vi "newTestStandStringVariable.vi"(0 "Engine Reference":refnum<k7>, 5 "Sequence File Ref":refnum<k7>, 7 "Variable Name":string="Locals.temp", 9 "Variable Value":string, 11 "error in":errorcluster) -> (4 "Engine Reference (out)":refnum<k7>, 6 "Sequence File (out)":refnum<k7>, 15 "error out":errorcluster)   [LabVIEW 2010]
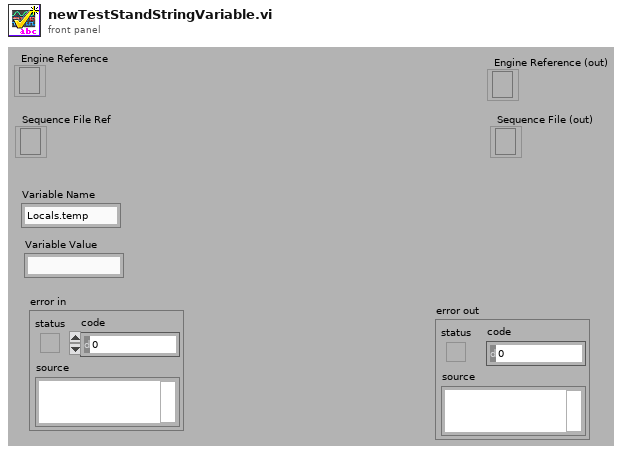
[diagram p1: front panel]
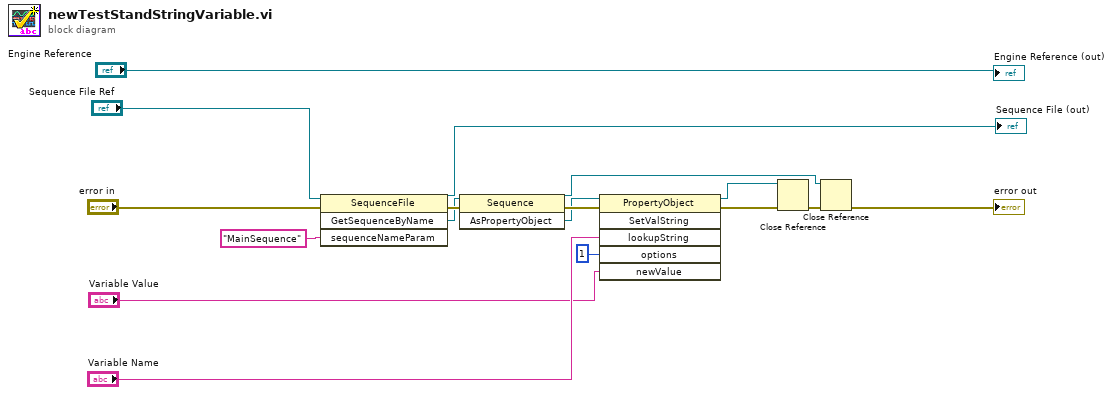
[diagram p0: block diagram]
diagram:
  n1 = invoke class="SequenceFile" method="GetSequenceByName"(reference="Sequence File Ref", error in="error in", "sequenceNameParam"="MainSequence") -> (reference out=→"Sequence File (out)":refnum<k7>, error out=w12:errorcluster, "GetSequenceByName"=w10:refnum<k7>)  [unwired: 1 in, 1 out]
  n2 = invoke class="Sequence" method="AsPropertyObject"(reference=w10, error in=w12) -> (reference out=w15:refnum<k7>, error out=w7:errorcluster, "AsPropertyObject"=w6:refnum<k7>)  [unwired: 1 in]
  n3 = invoke class="PropertyObject" method="SetValString"(reference=w6, error in=w7, "lookupString"="Variable Name", "options"=1, "newValue"="Variable Value") -> (reference out=w3:refnum<k7>, error out=w1:errorcluster)  [unwired: 1 in, 4 out]
  n4 = Close Reference(reference=w3, error in (no error)=w1) -> (error out=w14:errorcluster)
  n5 = Close Reference(reference=w15, error in (no error)=w14) -> (error out=→"error out":errorcluster)
  "Engine Reference (out)" <- "Engine Reference"
